vi "测试-探头模板.vi"() -> ()   [LabVIEW 2017]
panel:
  in  "枚举":enum16{"2~8模板-网络版", "12模板-网络版"}(ring)
  in  "等待时间（毫秒）":u32=500
  in  "停止按钮":bool
  in  "限值":cluster{"限值1":dbl, "限值2":dbl}={"限值1"=1.0, "限值2"=100.0}
  in  "最低水平":dbl=0.15 format="%#_13g"
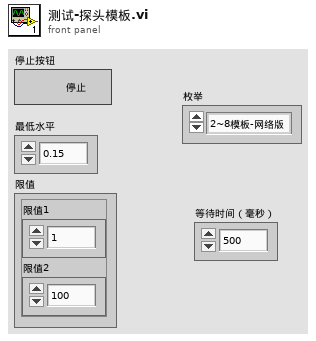
[diagram p1: front panel]
types:
  T1 = cluster{"探头地址与信息":cluster{"网络地址":cluster{"IP":string, "port":u16}, "探头信息":string}, "测量值":cluster{"时间":timestamp, "数值":dbl}, "限值":cluster{"限值1":dbl, "限值2":dbl}, "探头状态":enum16{"正常", "离线", "禁用", "一级报警", "二级报警"}}
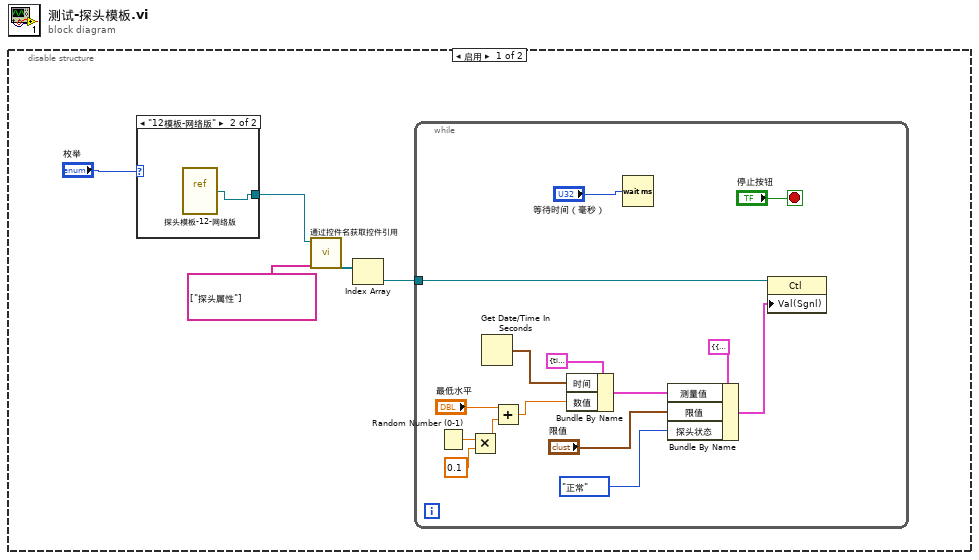
[diagram p0: block diagram]
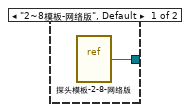
[diagram p2: hidden frame]
diagram:
  n1 = disable-structure shown="启用" {
    frame Enabled {
      n2 = case shown="\"12模板-网络版\"" "枚举" {
        tunnel: [w6 w7] -> w5
        frame "2~8模板-网络版", Default {
          n3 = vi-ref "探头模板-2-8-网络版.vi"() -> (w6:refnum<vi>)
        }
        frame "12模板-网络版" {
          n4 = vi-ref "探头模板-12-网络版.vi"() -> (w7:refnum<vi>)
        }
      }
      n5 = call "通过控件名获取控件引用.vi"("控件名数组"=string[] ["探头属性"], "VI引用"=w5) -> ("控件引用输出"=w3:refnum<vi>[])  [unwired: 7 in, 2 out]
      n6 = Index Array(array=w3) -> (element=w2:refnum<vi>)  [unwired: 1 in]
      n7 = while {
        tunnel: w2 -> [w22]
        stop <- "停止按钮" stop-if-true
        n8 = Random Number (0-1)() -> (number: 0 to 1=w19:dbl)
        n9 = Multiply(x=w19, y=0.1) -> (x*y=w9:dbl)
        n10 = Get Date/Time In Seconds() -> (seconds since 1Jan1904=w18:timestamp)
        n11 = Add(x="最低水平", y=w9) -> (x+y=w17:dbl)
        n12 = Bundle By Name(cluster=cluster{"时间":timestamp, "数值":dbl} {"时间"=timestamp(0 s since 1904-01-01), "数值"=0.0} ("测量值"), "时间"=w18, "数值"=w17) -> (w15:cluster{"时间":timestamp, "数值":dbl})
        n13 = Wait (ms)(milliseconds to wait="等待时间（毫秒）") -> ()  [unwired: 1 out]
        n14 = Bundle By Name(cluster=T1 {"探头地址与信息"={"网络地址"={"IP"="", "port"=0}, "探头信息"=""}, "测量值"={"时间"=timestamp(3554955153.6246996 s since 1904-01-01), "数值"=0.0}, "限值"={"限值1"=1.0, "限值2"=100.0}, "探头状态"=enum."正常"} ("探头属性"), "测量值"=w15, "限值"="限值", "探头状态"=enum16{"正常", "离线", "禁用", "一级报警", "二级报警"}."正常") -> (w12:T1)
        n15 = property class="Ctl"(reference=w22, "Val(Sgnl)"=w12) -> ()  [unwired: 1 in, 2 out]
      }
    }
    frame Disabled {
    }
  }
